vi "Write Element of V_SysV2.vi"(8 "error in (no error)":errorcluster, 9 "Numeric":dbl, 10 "index":i32, 11 "ChirpV2 in":refnum<class "ChirpV2.lvclass">) -> (0 "error out":errorcluster, 3 "ChirpV2 out":refnum<class "ChirpV2.lvclass">)   [LabVIEW 2014]
uses:
  ChirpV2.lvclass
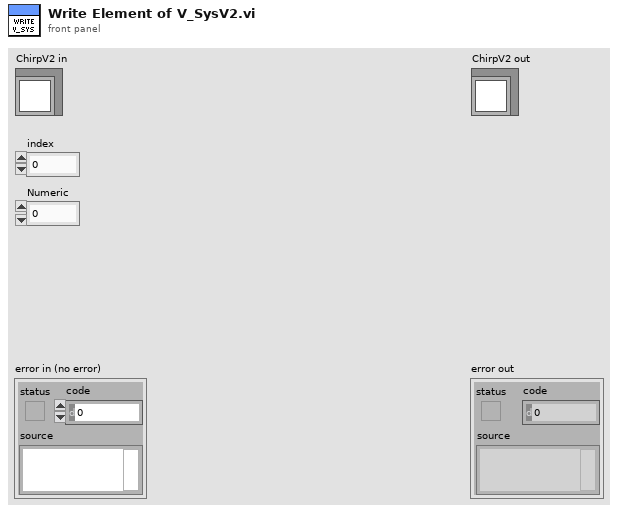
[diagram p1: front panel]
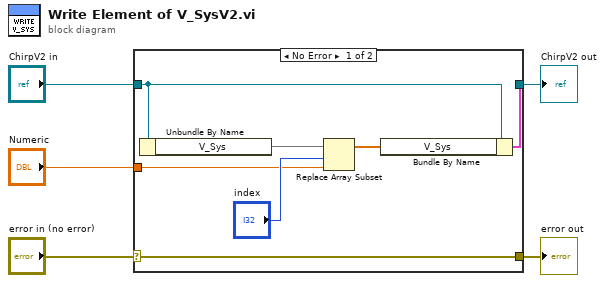
[diagram p0: block diagram]
diagram:
  n1 = case shown="No Error" "error in (no error)" {
    selector: "error in (no error)" -> [w12 w13]
    tunnel: [w12 w13] -> w4
    tunnel: [w11 w14] -> w2
    tunnel: "ChirpV2 in" -> [w10 w14]
    tunnel: "Numeric" -> [w6 _]
    frame No Error {
      n2 = Unbundle By Name(w10) -> ("V_Sys"=w9)
      n3 = Replace Array Subset(array=w9, new element=w6, index="index") -> (w8:dbl[])
      n4 = Bundle By Name(cluster=w10, "V_Sys"=w8) -> (w11:cluster{})
    }
    frame Error {
    }
  }
  "error out" <- w4
  "ChirpV2 out" <- w2
